vi "Destroy User Events_SM.vi"(8 "error in (no error)":errorcluster, 11 "Inspection Statemachine in":refnum<class "Inspection Statemachine.lvclass">) -> (0 "error out":errorcluster)   [LabVIEW 2019, in "Inspection Statemachine.lvclass"]
uses:
  Inspection Statemachine.lvclass
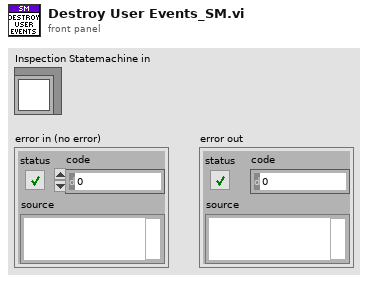
[diagram p1: front panel]
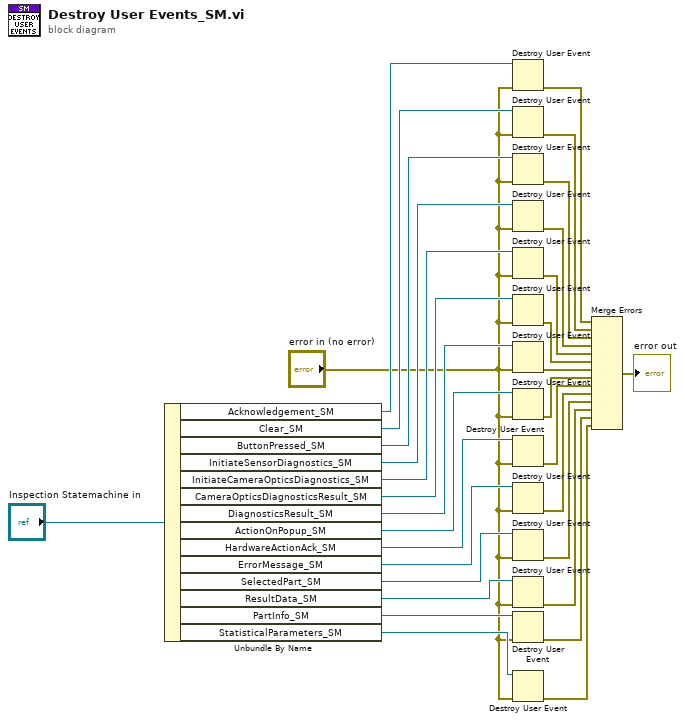
[diagram p0: block diagram]
diagram:
  n1 = Unbundle By Name("Inspection Statemachine in") -> ("Acknowledgement_SM"=w30:refnum<user-event>, "Clear_SM"=w29:refnum<user-event>, "ButtonPressed_SM"=w28:refnum<user-event>, "InitiateSensorDiagnostics_SM"=w27:refnum<user-event>, "InitiateCameraOpticsDiagnostics_SM"=w26:refnum<user-event>, "CameraOpticsDiagnosticsResult_SM"=w25:refnum<user-event>, "DiagnosticsResult_SM"=w24:refnum<user-event>, "ActionOnPopup_SM"=w23:refnum<user-event>, "HardwareActionAck_SM"=w22:refnum<user-event>, "ErrorMessage_SM"=w21:refnum<user-event>, "SelectedPart_SM"=w20:refnum<user-event>, "ResultData_SM"=w19:refnum<user-event>, "PartInfo_SM"=w18:refnum<user-event>, "StatisticalParameters_SM"=w17:refnum<user-event>)
  n2 = Destroy User Event(user event=w30, error in="error in (no error)") -> (error out=w15:errorcluster)
  n3 = Destroy User Event(user event=w29, error in="error in (no error)") -> (error out=w14:errorcluster)
  n4 = Destroy User Event(user event=w28, error in="error in (no error)") -> (error out=w13:errorcluster)
  n5 = Destroy User Event(user event=w27, error in="error in (no error)") -> (error out=w12:errorcluster)
  n6 = Destroy User Event(user event=w26, error in="error in (no error)") -> (error out=w11:errorcluster)
  n7 = Destroy User Event(user event=w25, error in="error in (no error)") -> (error out=w10:errorcluster)
  n8 = Destroy User Event(user event=w24, error in="error in (no error)") -> (error out=w9:errorcluster)
  n9 = Destroy User Event(user event=w23, error in="error in (no error)") -> (error out=w8:errorcluster)
  n10 = Destroy User Event(user event=w22, error in="error in (no error)") -> (error out=w7:errorcluster)
  n11 = Destroy User Event(user event=w21, error in="error in (no error)") -> (error out=w6:errorcluster)
  n12 = Destroy User Event(user event=w20, error in="error in (no error)") -> (error out=w5:errorcluster)
  n13 = Destroy User Event(user event=w19, error in="error in (no error)") -> (error out=w4:errorcluster)
  n14 = Destroy User Event(user event=w18, error in="error in (no error)") -> (error out=w3:errorcluster)
  n15 = Destroy User Event(user event=w17, error in="error in (no error)") -> (error out=w2:errorcluster)
  n16 = Merge Errors(w15, w14, w13, w12, w11, w10, w9, w8, w7, w6, w5, w4, w3, w2) -> (→"error out":errorcluster)
